vi "Configure Spectrum Emission Mask (Limit Setup).vi"(0 "VISA resource name":refnum<visa-resource-name>, 1 "SEM Abs Limit Start":dbl[](array[numeric]) min=-200.0 max=50.0 format="%.2f", 2 "SEM Abs Limit Stop":dbl[](array[numeric]) min=-200.0 max=50.0 format="%.2f", 5 "SEM Integer Level (0:Absolute Level 1)":i32(ring) items=["Absolute Level 1", "Absolute Level 2"], 7 "SEM Logic":i32[](array[ring]) items=["Not Judged (Off)", "Absolute Level Upper Limit 1", "Relative Level Upper Limit", "Absolute 1 AND Relative Level", "Absolute 1 OR Relative Level", "Absolute 1 AND Relative AND Absolute 2", "Absolute 1 OR Relative AND Absolute 2", "Absolute 1 AND Absolute 2 Level"], 11 "error in (no error)":errorcluster, 12 "SEM Limit Start":dbl[](array[numeric]) min=-200.0 max=50.0 format="%.2f", 13 "SEM Limit Stop":dbl[](array[numeric]) min=-200.0 max=50.0 format="%.2f") -> (4 "VISA resource name out":refnum<visa-resource-name>, 15 "error out":errorcluster)   [LabVIEW 2020, in "Anritsu Signal Analyzer Series.lvlib"]
doc: "Configures the Limit for SEM measurement"
uses:
  Anritsu Signal Analyzer Series.lvlib
panel:
  # "dBm"
  # "dB"
  # "dBm"
  # "dB"
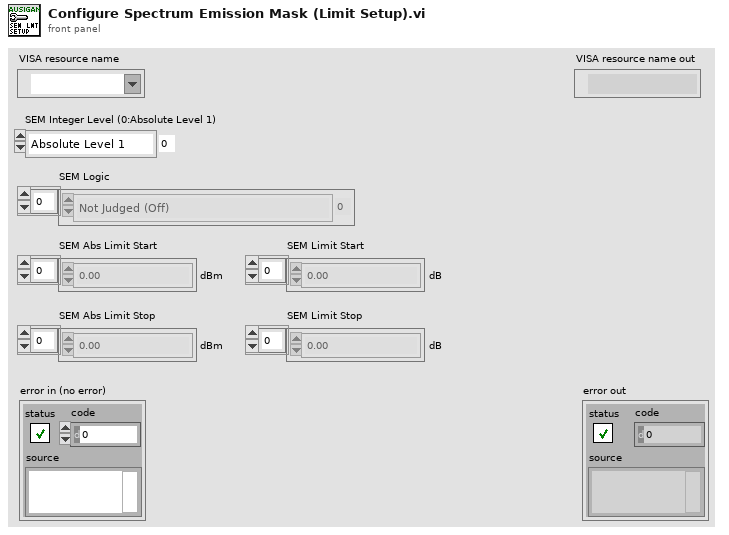
[diagram p1: front panel]
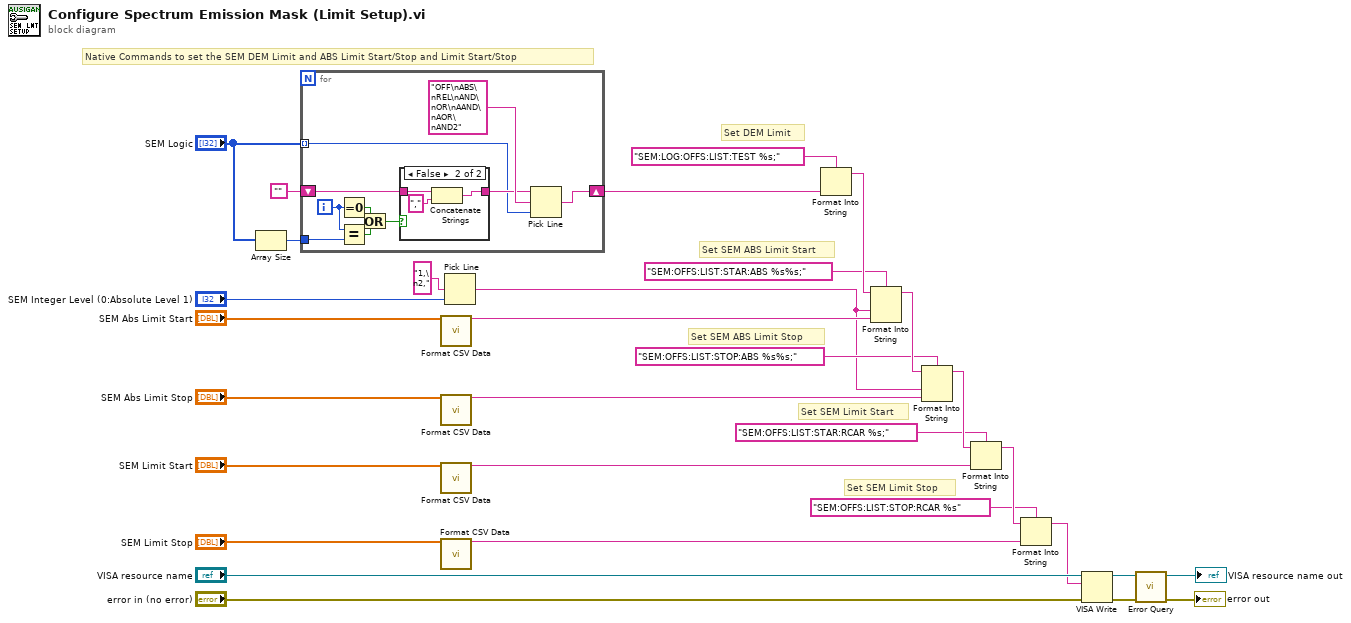
[diagram p0: block diagram]
diagram:
  # "Native Commands to set the SEM DEM Limit and ABS Limit Start/Stop and Limit Start/Stop"
  # "Set SEM Limit Stop"
  # "Set SEM Limit Start"
  # "Set SEM ABS Limit Stop"
  # "Set SEM ABS Limit Start"
  # "Set DEM Limit"
  n1 = Array Size(array="SEM Logic") -> (size(s)=w3:i32)
  n2 = for {
    shift-right: [w32] -> w20
    shift-left: "" -> [w41]
    tunnel: "SEM Logic" -> [w33] mode=indexing
    tunnel: w3 -> [w37]
    i -> [w38]
    n3 = Equal To 0?(x=w38) -> (x = 0?=w39:bool)
    n4 = Equal?(x=w38, y=w37) -> (x = y?=w40:bool)
    n5 = Or(x=w39, y=w40) -> (x .or. y?=w36:bool)
    n6 = case shown="False" w36 {
      tunnel: w41 -> [w42 w45]
      tunnel: [w42 w43] -> w34
      frame True {
      }
      frame False {
        n7 = Concatenate Strings(w45, "," ("string")) -> (w43:string)
      }
    }
    n8 = Pick Line(string ("")=w34, multi-line string="OFF\nABS\nREL\nAND\nOR\nAAND\nAOR\nAND2" ("複数行文字列"), line index=w33) -> (output string=w32:string)
  }
  n9 = call "Format CSV Data.vi"("Data_In"="SEM Abs Limit Start") -> ("Data_out"=w17:string)  [unwired: 14 in]
  n10 = call "Format CSV Data.vi"("Data_In"="SEM Abs Limit Stop") -> ("Data_out"=w14:string)  [unwired: 14 in]
  n11 = call "Format CSV Data.vi"("Data_In"="SEM Limit Start") -> ("Data_out"=w12:string)  [unwired: 14 in]
  n12 = call "Format CSV Data.vi"("Data_In"="SEM Limit Stop") -> ("Data_out"=w9:string)  [unwired: 14 in]
  n13 = Pick Line(multi-line string="1,\n2," ("複数行文字列"), line index="SEM Integer Level (0:Absolute Level 1)") -> (output string=w1:string)  [unwired: 1 in]
  n14 = Format Into String(format string="SEM:LOG:OFFS:LIST:TEST %s;" ("_CommandSet"), w20) -> (resulting string=w18:string)  [unwired: 2 in, 1 out]
  n15 = Format Into String(format string="SEM:OFFS:LIST:STAR:ABS %s%s;" ("_CommandSet"), initial string=w18, w1, w17) -> (resulting string=w15:string)  [unwired: 1 in, 1 out]
  n16 = Format Into String(format string="SEM:OFFS:LIST:STOP:ABS %s%s;" ("_CommandSet"), initial string=w15, w1, w14) -> (resulting string=w11:string)  [unwired: 1 in, 1 out]
  n17 = Format Into String(format string="SEM:OFFS:LIST:STAR:RCAR %s;" ("_CommandSet"), initial string=w11, w12) -> (resulting string=w8:string)  [unwired: 1 in, 1 out]
  n18 = Format Into String(format string="SEM:OFFS:LIST:STOP:RCAR %s" ("_CommandSet"), initial string=w8, w9) -> (resulting string=w6:string)  [unwired: 1 in, 1 out]
  n19 = VISA Write(VISA resource name="VISA resource name", write buffer=w6, error in (no error)="error in (no error)") -> (VISA resource name out=w5:refnum<visa-resource-name>, error out=w4:errorcluster)  [unwired: 1 out]
  n20 = call "Error Query.vi"("error in (no error)"=w4, "VISA resource name"=w5) -> ("error out"=→"error out":errorcluster, "VISA resource name out"=→"VISA resource name out":refnum<visa-resource-name>)  [unwired: 6 in, 2 out]
